vi "Ports To System Definition.vi"(8 "error in":errorcluster, 9 "ports":T2[](array[typedef]), 10 "parameter configuration file path":path, 11 "custom device ref":T1 format="%.0x") -> (0 "error out":errorcluster, 3 "custom device ref out":T1 format="%.0x")   [LabVIEW 2020, in "AIM ARINC 429 Scripting.lvlib"]
uses:
  AIM ARINC 429 Scripting.lvlib
  <vilib>/NI VeriStand/Custom Device API/Custom Device Item Ref.ctl
  <vilib>/NI VeriStand/Custom Device API/Custom Device API.lvlib
  <vilib>/NI/NI VeriStand Encoding and Decoding/Encoding.ctl
  <vilib>/NI/NI VeriStand Encoding and Decoding/Encoding and Decoding.lvlib
  Shared/Parameter Definition.ctl
  Shared/Direction.ctl
  Shared/VS Channel Definition for Parameter.ctl
  Shared/VS Channels Definition for Label.ctl
  Shared/VS Channels Definition for All Labels on Hardware Channel.ctl
  Shared/Transfer Type.ctl
  Shared/Transfer Speed.ctl
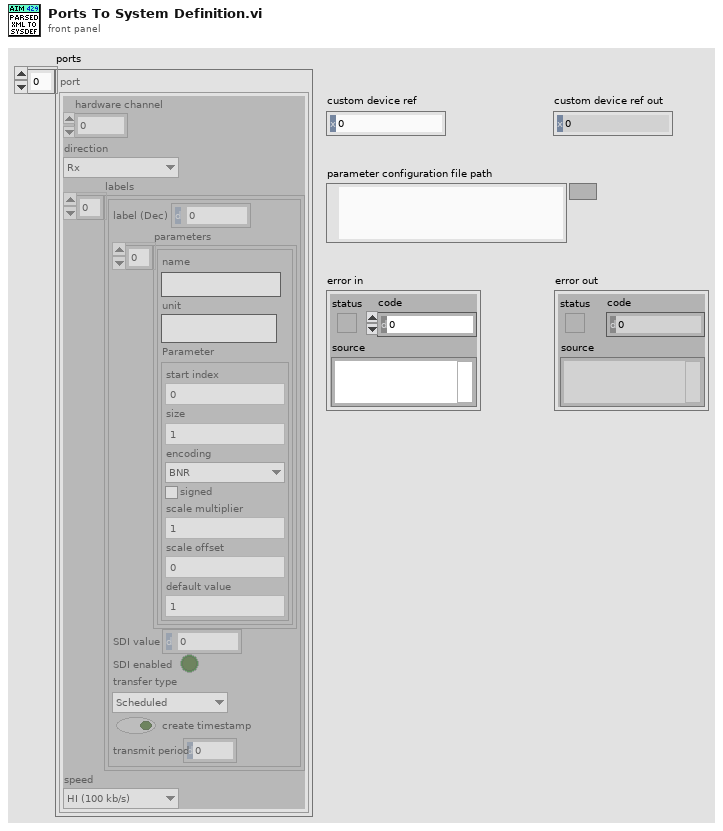
[diagram p1: front panel]
types:
  T1 = typedef "Custom Device API.lvlib/Custom Device Item Ref.ctl" = u64
  T2 = typedef "VS Channels Definition for All Labels on Hardware Channel.ctl" = cluster{"hardware channel":i32, "direction":T3, "labels":T4[], "speed":T9}
  T3 = typedef "Direction.ctl" = enum16{"Rx", "Tx"}
  T4 = typedef "VS Channels Definition for Label.ctl" = cluster{"label (Dec)":u32, "parameters":T5[], "SDI value":u8, "SDI enabled":bool, "transfer type":T8, "create timestamp":bool, "transmit period":u32}
  T5 = typedef "VS Channel Definition for Parameter.ctl" = cluster{"name":string, "unit":string, "Parameter":T6}
  T6 = typedef "Parameter Definition.ctl" = cluster{"start index":i32, "size":i32, "encoding":T7, "signed":bool, "scale multiplier":dbl, "scale offset":dbl, "default value":dbl}
  T7 = typedef "Encoding and Decoding.lvlib/Encoding.ctl" = enum16{"BNR", "BCD", "Discrete"}
  T8 = typedef "Transfer Type.ctl" = enum16{"Scheduled", "Acyclic", "Block", "Strobe"}
  T9 = typedef "Transfer Speed.ctl" = enum16{"LO (12.5 kb/s)", "HI (100 kb/s)"}
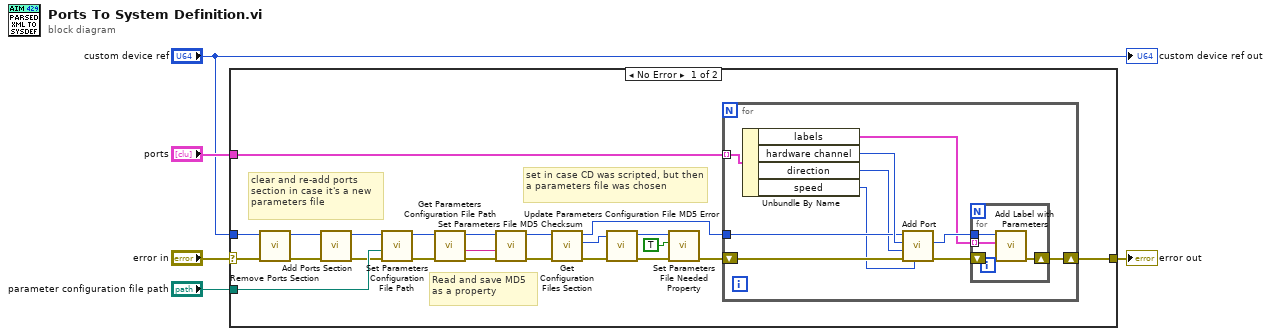
[diagram p0: block diagram]
diagram:
  n1 = case shown="No Error" "error in" {
    selector: "error in" -> [w24 w43]
    tunnel: "custom device ref" -> [w25 _]
    tunnel: [w28 w43] -> w5
    tunnel: "ports" -> [w27 _]
    tunnel: "parameter configuration file path" -> [w26 _]
    frame No Error {
      # "set in case CD was scripted, but then a parameters file was chosen"
      # "Read and save MD5 as a property"
      # "clear and re-add ports section in case it's a new parameters file"
      n2 = call "Remove Ports Section.vi"("error in"=w24, "custom device ref"=w25) -> ("error out"=w23:errorcluster, "custom device ref out"=w22:T1)  [unwired: 8 in]
      n3 = call "Add Ports Section.vi"("error in"=w23, "custom device ref"=w22) -> ("error out"=w20:errorcluster, "custom device ref out"=w21:T1)  [unwired: 7 in, 1 out]
      n4 = call "Set Parameters Configuration File Path.vi"("error in"=w20, "parameters configuration file path"=w26, "AIM ARINC 429 custom device in"=w21) -> ("error out"=w10:errorcluster, "AIM ARINC 429 custom device out"=w9:T1)  [unwired: 7 in]
      n5 = call "Get Parameters Configuration File Path.vi"("error in"=w10, "AIM ARINC 429 custom device in"=w9) -> ("error out"=w18:errorcluster, "MD5 checksum"=w17:string, "AIM ARINC 429 custom device  out"=w19:T1)  [unwired: 6 in, 1 out]
      n6 = call "Set Parameters File MD5 Checksum.vi"("error in"=w18, "MD5"=w17, "custom device ref"=w19) -> ("error out"=w15:errorcluster, "custom device ref out"=w16:T1)  [unwired: 7 in]
      n7 = call "Get Configuration Files Section.vi"("error in"=w15, "Custom device Ref"=w16) -> ("error out"=w14:errorcluster, "Configuration files Ref"=w13:T1, "Custom device Ref out"=w12:T1)  [unwired: 7 in]
      n8 = call "Update Parameters Configuration File MD5 Error.vi"("error in"=w14, "configuration files ref"=w13) -> ("error out"=w8:errorcluster, "configuration files ref out"=w6:T1)  [unwired: 8 in]
      n9 = call "Set Parameters File Needed Property.vi"("error in"=w8, "needed"=TRUE, "configuration files ref"=w6) -> ("error out"=w7:errorcluster)  [unwired: 7 in, 1 out]
      n10 = for {
        shift-right: [w35] -> w28
        shift-left: w7 -> [w32]
        tunnel: w12 -> [w33]
        tunnel: w27 -> [w38] mode=indexing
        n11 = Unbundle By Name(w38) -> ("labels"=w31:T4[], "hardware channel"=w34:i32, "direction"=w30:T3, "speed"=w29:T9)
        n12 = call "Add Port.vi"("speed"=w29, "error in"=w32, "direction"=w30, "port number"=w34, "AIM ARINC 429 custom device in"=w33) -> ("error out"=w37:errorcluster, "port"=w36:T1)  [unwired: 4 in, 1 out]
        n13 = for {
          tunnel: w36 -> [w41]
          tunnel: w31 -> [w39] mode=indexing
          shift-right: [w40] -> w35
          shift-left: w37 -> [w42]
          n14 = call "Add Label with Parameters.vi"("error in"=w42, "label"=w39, "port ref"=w41) -> ("error out"=w40:errorcluster)  [unwired: 7 in, 1 out]
        }
      }
    }
    frame Error {
    }
  }
  "error out" <- w5
  "custom device ref out" <- "custom device ref"
